vi "get Power-on Status Clear.vi"(8 "error in (no error)":errorcluster, 11 "VISA resource name":refnum<visa-resource-name>) -> (0 "error out":errorcluster, 2 "Power-on Status Flag":bool, 3 "VISA resource name out":refnum<visa-resource-name>, 4 "Device Errors":cluster{"code":i32, "Text":string}[](array[cluster]))   [LabVIEW 2014, in "Stanford Research DG645 - Driver.lvlib"]
doc: "Common IEEE-488.2 Command: *PSC?\nInstrument Error Check\n\nQuery the Power-on Status Clear flag. If the value on the flag is false, then the Service Request Enable and Standard Event Status Enable Registers (*SRE, *ESE) are stored in non-volontile memory, and retain their values through power-cycle events. If the value of the flag is true, then these two registers are cleared upon power-cycle."
uses:
  Stanford Research DG645 - Driver.lvlib
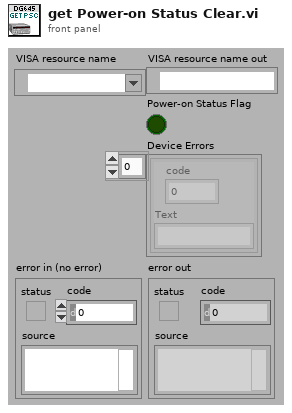
[diagram p1: front panel]
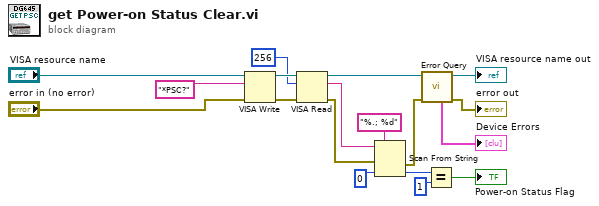
[diagram p0: block diagram]
diagram:
  n1 = VISA Write(VISA resource name="VISA resource name", write buffer="*PSC?" ("command"), error in (no error)="error in (no error)") -> (VISA resource name out=w16:refnum<visa-resource-name>, error out=w15:errorcluster)  [unwired: 1 out]
  n2 = VISA Read(VISA resource name=w16, byte count=u32 256, error in (no error)=w15) -> (VISA resource name out=w5:refnum<visa-resource-name>, read buffer=w12:string, error out=w10:errorcluster)  [unwired: 1 out]
  n3 = Scan From String(format string="%.; %d", input string=w12, error in=w10, default 1=0 ("default value 1")) -> (error out=w3:errorcluster, output 1=w8:i32)  [unwired: 1 in, 2 out]
  n4 = call "Error Query.vi"("error in (no error)"=w3, "VISA resource name"=w5) -> ("error out"=→"error out":errorcluster, "VISA resource name out"=→"VISA resource name out":refnum<visa-resource-name>, "Device Errors"=→"Device Errors":cluster{"code":i32, "Text":string}[])  [unwired: 7 in]
  n5 = Equal?(x=w8, y=1) -> (x = y?=→"Power-on Status Flag":bool)
